vi "controlReferenceAutoUpdate.vi"(7 "Set":bool, 8 "error in":errorcluster, 9 "ref auto up in":bool=TRUE, 10 "axis in":u8, 11 "connection ID":refnum<k5>) -> (0 "error out":errorcluster, 1 "ref auto up out":bool=TRUE, 2 "axis out":u8, 3 "connection ID":refnum<k5>)   [LabVIEW 2019]
panel:
  in  "Set Command":string="com.attocube.amc.control.setControlReferenceAutoUpdate"
  in  "Get Command":string="com.attocube.amc.control.getControlReferenceAutoUpdate"
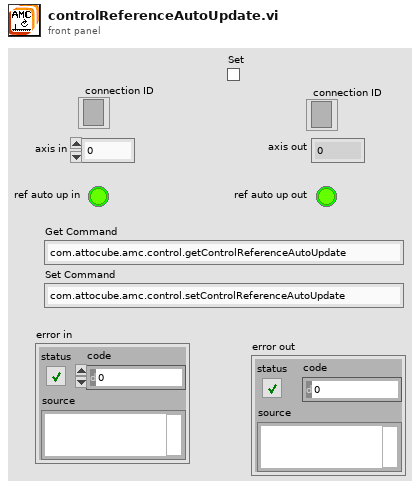
[diagram p1: front panel]
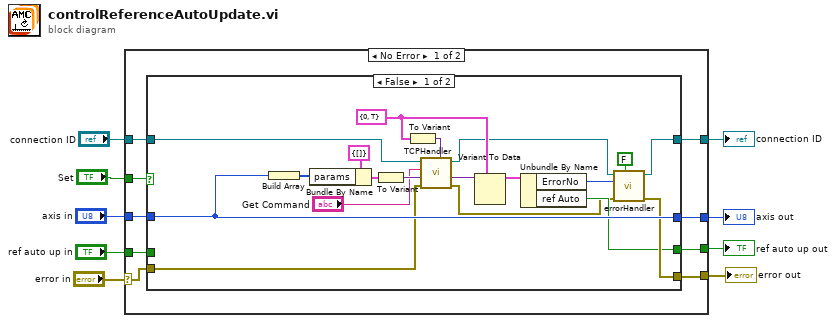
[diagram p0: block diagram]
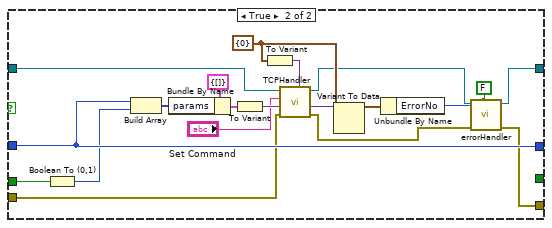
[diagram p2: hidden frame]
diagram:
  n1 = case shown="No Error" "error in" {
    selector: "error in" -> [w10 w61]
    tunnel: "axis in" -> [w16 w59]
    tunnel: [w11 w61] -> w8
    tunnel: [w13 w59] -> w7
    tunnel: "Set" -> [w17 _]
    tunnel: "ref auto up in" -> [w15 w60]
    tunnel: [w14 w58] -> w4
    tunnel: "connection ID" -> [w18 w58]
    tunnel: [w12 w60] -> w2
    frame No Error {
      n2 = case shown="False" w17 {
        tunnel: [w22 w41] -> w14
        tunnel: w18 -> [w27 w52]
        tunnel: w16 -> [w29 w50]
        tunnel: [w29 w50] -> w13
        tunnel: [w28 w47] -> w11
        tunnel: [w24 _] -> w12
        tunnel: w15 -> [_ w43]
        tunnel: w10 -> [w20 w39]
        frame False {
          w25 = cluster{"ErrorNo":i16, "ref Auto":bool} {"ErrorNo"=0, "ref Auto"=TRUE} ("input cluster")
          n3 = Build Array(w29) -> (w33:u8[])
          n4 = Bundle By Name(cluster=cluster{"params":i16[]} {"params"=[]} ("input cluster"), "params"=w33) -> (w34:cluster{"params":i16[]})
          n5 = To Variant(anything=w34) -> (Variant=w35:variant)
          n6 = To Variant(anything=w25) -> (Variant=w26:variant)
          n7 = call <userlib>:"TCPHandler.vi"("result Types"=w26, "error in (no error)"=w20, "params"=w35, "method"="Get Command", "connection ID"=w27) -> ("error out"=w19:errorcluster, "result"=w31:variant, "connection ID"=w23:refnum<k5>)  [unwired: 3 in, 1 out]
          n8 = Variant To Data(type=w25, Variant=w31) -> (data=w36:cluster{"ErrorNo":i16, "ref Auto":bool})  [unwired: 1 in, 1 out]
          n9 = Unbundle By Name(w36) -> ("ErrorNo"=w37:i16, "ref Auto"=w24:bool)
          n10 = call <userlib>:"errorHandler.vi"("show popup"=FALSE, "error in"=w19, "error number"=w37, "connection ID"=w23) -> ("error out"=w28:errorcluster, "connection ID"=w22:refnum<k5>)  [unwired: 6 in]
        }
        frame True {
          w45 = cluster{"ErrorNo":i16} {"ErrorNo"=0} ("input cluster")
          n11 = Boolean To (0,1)(Boolean=w43) -> (0, 1=w44:i16)
          n12 = Build Array(w50, w44) -> (w54:i16[])
          n13 = Bundle By Name(cluster=cluster{"params":i64[]} {"params"=[]} ("input cluster"), "params"=w54) -> (w53:cluster{"params":i64[]})
          n14 = To Variant(anything=w53) -> (Variant=w51:variant)
          n15 = To Variant(anything=w45) -> (Variant=w46:variant)
          n16 = call <userlib>:"TCPHandler.vi"("result Types"=w46, "error in (no error)"=w39, "params"=w51, "method"="Set Command", "connection ID"=w52) -> ("error out"=w38:errorcluster, "result"=w56:variant, "connection ID"=w42:refnum<k5>)  [unwired: 3 in, 1 out]
          n17 = Variant To Data(type=w45, Variant=w56) -> (data=w49:cluster{"ErrorNo":i16})  [unwired: 1 in, 1 out]
          n18 = Unbundle By Name(w49) -> ("ErrorNo"=w48:i16)
          n19 = call <userlib>:"errorHandler.vi"("show popup"=FALSE, "error in"=w38, "error number"=w48, "connection ID"=w42) -> ("error out"=w47:errorcluster, "connection ID"=w41:refnum<k5>)  [unwired: 6 in]
        }
      }
    }
    frame Error {
    }
  }
  "error out" <- w8
  "axis out" <- w7
  "ref auto up out" <- w2
  "connection ID" <- w4
